vi "Get Instrument Info.vi"(0 "NI-568x Power Meter in":refnum<class "Power Meter.lvclass">, 11 "error in":errorcluster) -> (4 "NI-568x Power Meter out":refnum<class "Power Meter.lvclass">, 15 "error out":errorcluster)   [LabVIEW 2023, in "NI-568x RF Power Meter.lvlib" / "Power Meter.lvclass"]
uses:
  Power Meter.lvclass
  C:/srd-semi-rfcal-software/AuxTools/STSRFFixtureCharactUtility/Source/Code Modules/Fixture/Instruments/Power Meter/Power Meter Base/Power Meter Base.lvclass
  Instruments/Power Meter/Power Meter Base/Type Definitions/Instrument Info.ctl
  Instruments/Power Meter/Power Meter Base/Power Meter Base.lvclass/Power Meter Base.ctl
  Instruments/Power Meter/Power Meter Base/Properties/Write Instrument Info Array.vi
  <vilib>/nisyscfg/Find Hardware.vi
  <vilib>/nisyscfg/Close (System).vi
  <resource>/objmgr/rfSysapiTags.rc
  <vilib>/nisyscfg/nisyscfg.lvlib
  Instruments/Power Meter/Power Meter Base/Power Meter Base.lvclass
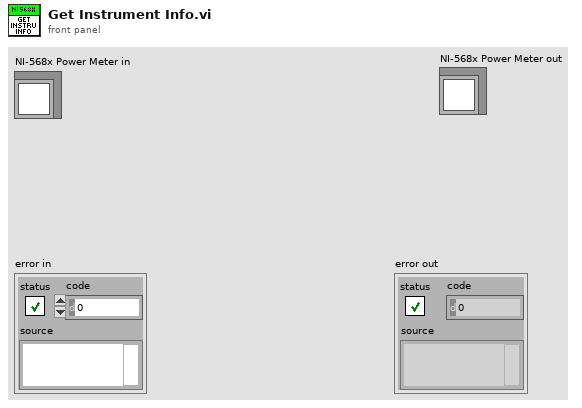
[diagram p1: front panel]
types:
  T1 = typedef "RFFixtureCharact.Instruments.lvlib/Power Meter Base.lvclass/Instrument Info.ctl" = cluster{"User Alias":string, "Resource Name":string, "Product Name":string, "Vendor Name":string}
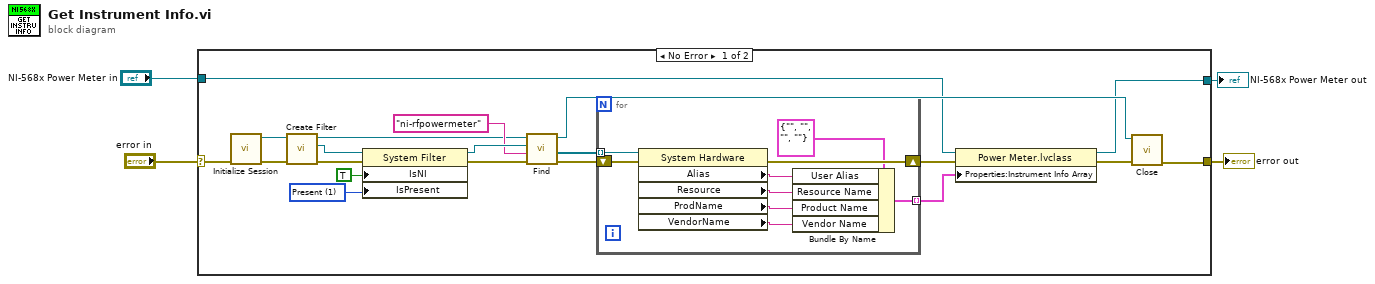
[diagram p0: block diagram]
diagram:
  n1 = case shown="No Error" "error in" {
    selector: "error in" -> [w15 w35]
    tunnel: [w11 w35] -> w3
    tunnel: "NI-568x Power Meter in" -> [w8 w34]
    tunnel: [w6 w34] -> w1
    frame No Error {
      w14 = 1 items=["Unknown"=-1, "Not Present"=0, "Present"=1] ("Devices & Chassis:Is Present")
      n2 = call <vilib>:"Initialize Session.vi"("error in (no error)"=w15) -> ("error out"=w19:errorcluster, "Session out"=w21:refnum<k21>)  [unwired: 9 in]
      n3 = call <vilib>:"Create Filter.vi"("error in (no error)"=w19, "Session in"=w21) -> ("error out"=w24:errorcluster, "Filter out"=w16:refnum<k20>, "Session out"=w17:refnum<k21>)  [unwired: 7 in]
      n4 = property class="System Filter"(reference=w16, error in=w24, "IsNI"=TRUE ("Devices & Chassis:Is NI Product"), "IsPresent"=w14) -> (reference out=w23:refnum<k20>, error out=w22:errorcluster)
      n5 = call-poly <vilib>:"Find.vi"("error in (no error)"=w22, "Experts"="ni-rfpowermeter", "Filter in"=w23, "Session in"=w17) -> ("error out"=w13:errorcluster, "Resources out"=w12:refnum<k20>[], "Session out"=w10:refnum<k21>)  [unwired: 4 in, 1 out]
      n6 = for {
        tunnel: w12 -> [w33] mode=indexing
        shift-right: [w32] -> w7
        shift-left: w13 -> [w31]
        tunnel: [w25] -> w5 mode=indexing
        n7 = property class="System Hardware"(reference=w33, error in=w31) -> (error out=w32:errorcluster, "Alias"=w30:string, "Resource"=w29:string, "ProdName"=w28:string, "VendorName"=w27:string)  [unwired: 1 out]
        n8 = Bundle By Name(cluster=T1 {"User Alias"="", "Resource Name"="", "Product Name"="", "Vendor Name"=""} ("Instrument Info Cluster"), "User Alias"=w30, "Resource Name"=w29, "Product Name"=w28, "Vendor Name"=w27) -> (w25:T1)
      }
      n9 = property class="Power Meter.lvclass"(reference=w8, error in=w7, "Properties:Instrument Info Array"=w5) -> (reference out=w6:refnum<class "Power Meter.lvclass">, error out=w9:errorcluster)
      n10 = call-poly <vilib>:"Close.vi"("error in (no error)"=w9, "Session in"=w10) -> ("error out"=w11:errorcluster)  [unwired: 9 in]
    }
    frame Error {
    }
  }
  "error out" <- w3
  "NI-568x Power Meter out" <- w1
